vi "Main.vi"(11 "Module Admin":refnum<class "Delacor_lib_QMH_Module Admin.lvclass">) -> ()   [LabVIEW 2020, in "Wordle Engine.lvlib"]
doc: "This template is based off of the Queued Message Handler design pattern and the Queued Message Handler project template that ships with LabVIEW.\n\nThe main difference is that the queue is private to this module and communication between modules is performed via Broadcast and Request events.\n\nRequest events are wrapped in public API methods and are handled in the Event Handling Loop (EHL) of this VI. Any module can register for Broadcast events sent by this module. The EHL generates messages based on user interface actions.\n\nThe Message Handling Loop (MHL) processes messages generated by the EHL, or by other messages. The messages are string values, so new messages can be added easily to the Message Cases case structure in the MHL. Each message cluster can also provide an optional value for Message Data, which is a variant that can be converted to whatever message-specific data is required.\n_____\nBased on DQMH Project Template 6.1.0.93."
uses:
  Wordle Engine.lvlib
  <vilib>/Delacor/Delacor QMH/Libraries/Module Admin_class/Delacor_lib_QMH_Module Admin.lvclass
  Module Data--cluster.ctl
  Stop Argument--cluster.ctl
  <vilib>/Delacor/Delacor QMH/Libraries/Message Queue_class/Delacor_lib_QMH_Message Queue.lvclass/Delacor_lib_QMH_Message Queue.ctl
  <vilib>/Delacor/Delacor QMH/Libraries/Module Admin_class/Delacor_lib_QMH_Module Admin.lvclass/Delacor_lib_QMH_Module Admin.ctl
  Select New Word Argument--cluster.ctl
  Select New Word (Reply Payload)--cluster.ctl
  Make a Guess Argument--cluster.ctl
  Make a Guess (Reply Payload)--cluster.ctl
  Apply Solver Argument--cluster.ctl
  Apply Solver (Reply Payload)--cluster.ctl
  Debug - Solve Specific Word Argument--cluster.ctl
  Debug - Solve Specific Word (Reply Payload)--cluster.ctl
  <vilib>/Delacor/Delacor QMH/Libraries/Message Queue_class/Delacor_lib_QMH_Enqueue Message (Single).vi
  <vilib>/Delacor/Delacor QMH/Libraries/Module Admin_class/Delacor_lib_QMH_Get External Launch.vi
  <vilib>/Utility/error.llb/Error Cluster From Error Code.vi
  <vilib>/ErrorRing/Error Ring.xnode
  <vilib>/Delacor/Delacor QMH/Libraries/Message Queue_class/Delacor_lib_QMH_Message Queue.lvclass
panel:
  out "error out":errorcluster
  # "This is a headless module."
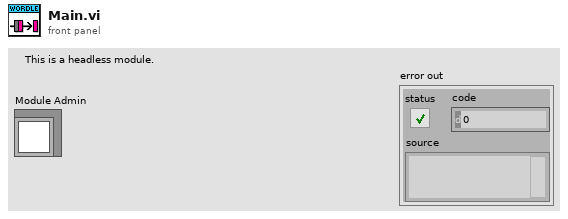
[diagram p1: front panel]
types:
  T1 = typedef "Wordle Engine.lvlib/Request Events--cluster.ctl" = cluster{"Stop Module":refnum<user-event>, "Show Panel":refnum<user-event>, "Hide Panel":refnum<user-event>, "Get Module Execution Status":refnum<user-event>, "Show Diagram":refnum<user-event>, "Select New Word":refnum<user-event>, "Make a Guess":refnum<user-event>, "Apply Solver":refnum<user-event>, "Debug - Solve Specific Word":refnum<user-event>}
  T2 = typedef "Wordle Engine.lvlib/Module Data--cluster.ctl" = cluster{"Used Words":set{string}, "Current Word":string}
  T3 = enum32{"invalid lock state", "Not Locked", "Locked (No Password)", "Password-protected"}
  T4 = typedef "Wordle Engine.lvlib/Stop Argument--cluster.ctl" = cluster{"Origin":string, "Exit via Stop Module Req?":bool, "Wait for Module to stop?":bool}
  T5 = typedef "Wordle Engine.lvlib/Select New Word Argument--cluster.ctl" = cluster{"Exclude Previously Selected Words":bool, "Wait Notifier":refnum<notifier>, "wait for reply":bool}
  T6 = typedef "Wordle Engine.lvlib/Make a Guess Argument--cluster.ctl" = cluster{"Guess":string, "Wait Notifier":refnum<notifier>, "wait for reply":bool}
  T7 = typedef "Wordle Engine.lvlib/Apply Solver Argument--cluster.ctl" = cluster{"Solver VI":path, "Number of Runs (1)":i32, "Wait Notifier":refnum<notifier>, "wait for reply":bool}
  T8 = typedef "Wordle Engine.lvlib/Debug - Solve Specific Word Argument--cluster.ctl" = cluster{"Word to Solve":string, "Solver VI":path, "Wait Notifier":refnum<notifier>, "wait for reply":bool}
  T9 = typedef "Wordle Engine.lvlib/Select New Word (Reply Payload)--cluster.ctl" = cluster{"New Word":string, "error":errorcluster}
  T10 = typedef "Wordle Engine.lvlib/Make a Guess (Reply Payload)--cluster.ctl" = cluster{"Result":string, "error":errorcluster}
  T11 = typedef "Wordle Engine.lvlib/Apply Solver (Reply Payload)--cluster.ctl" = cluster{"Average Solve Count":dbl, "Detailed Results":string, "error":errorcluster}
  T12 = typedef "Wordle Engine.lvlib/Debug - Solve Specific Word (Reply Payload)--cluster.ctl" = cluster{"Results":string, "error":errorcluster}
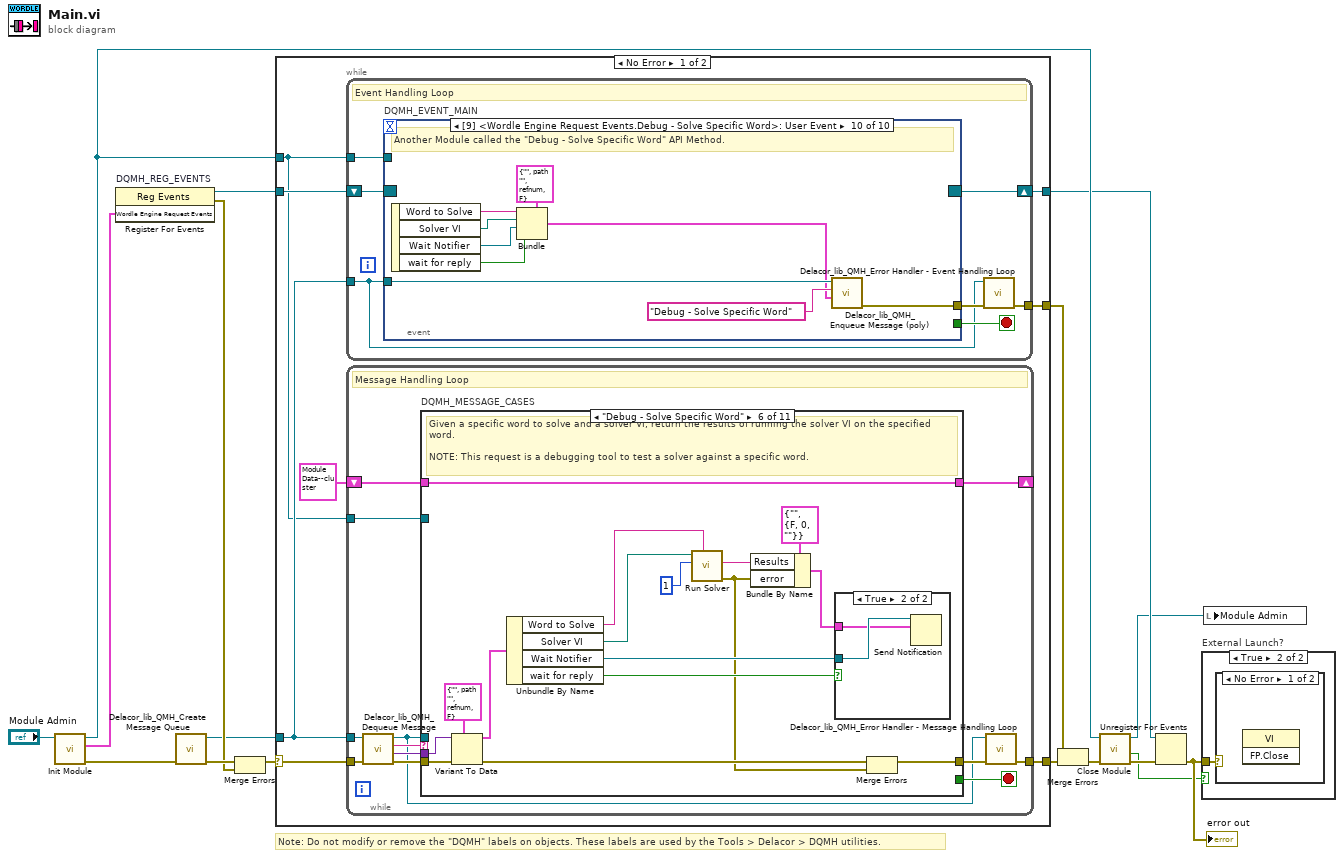
[diagram p0: block diagram]
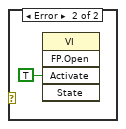
[diagram p3: hidden frame]
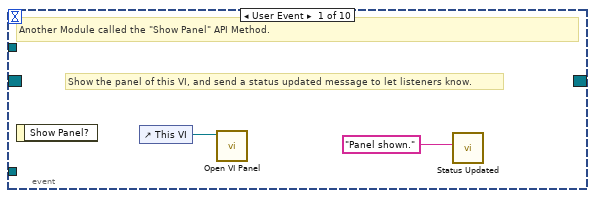
[diagram p4: hidden frame]
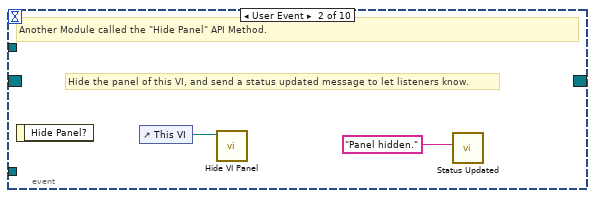
[diagram p5: hidden frame]
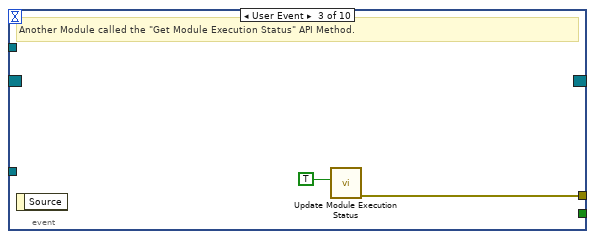
[diagram p6: hidden frame]
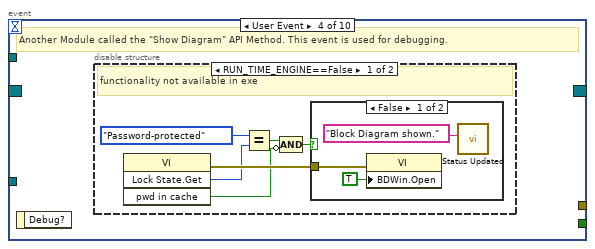
[diagram p7: hidden frame]
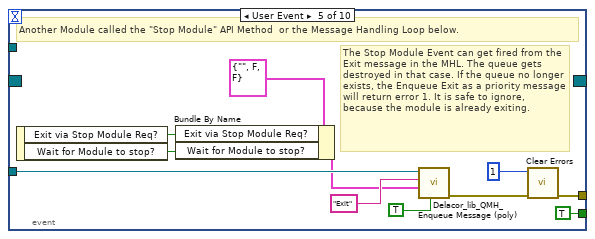
[diagram p10: hidden frame]
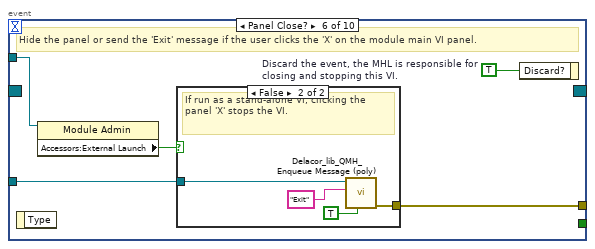
[diagram p11: hidden frame]
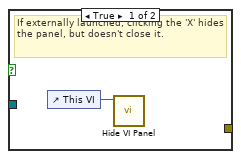
[diagram p12: hidden frame]
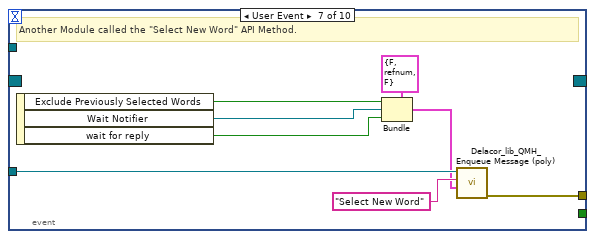
[diagram p13: hidden frame]
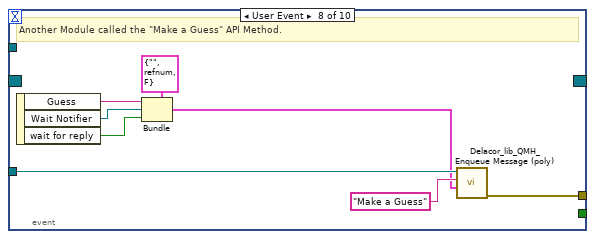
[diagram p14: hidden frame]
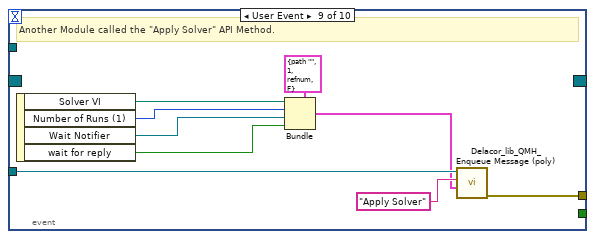
[diagram p15: hidden frame]
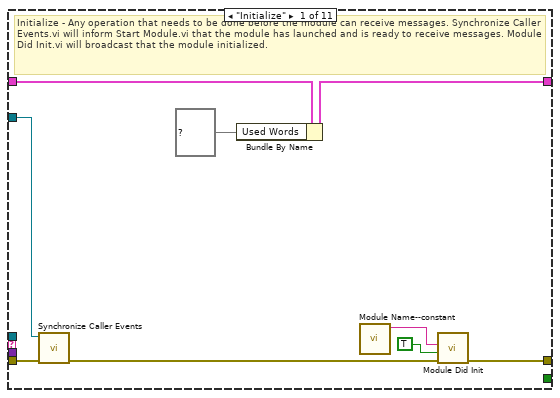
[diagram p16: hidden frame]
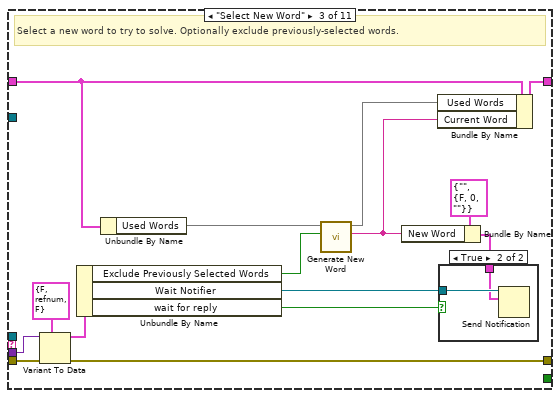
[diagram p18: hidden frame]
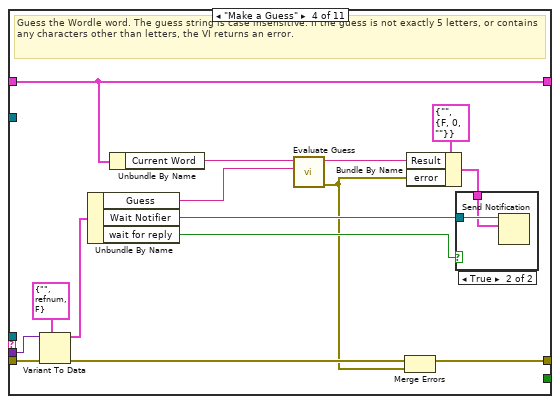
[diagram p20: hidden frame]
diagram:
  # "Note: Do not modify or remove the \"DQMH\" labels on objects. These labels are used by the Tools > Delacor > DQMH utilities."
  n1 = call "Init Module.vi"("Singleton Module Admin in"="Module Admin") -> ("error out"=w16:errorcluster, "Wordle Engine Request Events"=w5:T1, "Singleton Module Admin out"=w8:refnum<class "Delacor_lib_QMH_Module Admin.lvclass">)  [unwired: 8 in]
  n2 = register-events "DQMH_REG_EVENTS"(w5) -> (reference out=w6:refnum<event-registration>, error out=w9:errorcluster)  [unwired: 2 in]
  n3 = call <vilib>:"Delacor_lib_QMH_Create Message Queue.vi"("error in"=w16) -> ("error out"=w11:errorcluster, "Message Queue"=w4:refnum<class "Delacor_lib_QMH_Message Queue.lvclass">)  [unwired: 9 in]
  n4 = Merge Errors(w11, w9) -> (w10:errorcluster)
  n5 = case shown="No Error" w10 {
    selector: w10 -> [w23 w248]
    tunnel: [w25 w247] -> w17
    tunnel: [w22 w253] -> w7
    tunnel: w6 -> [w20 w253]
    tunnel: w4 -> [w19 w246]
    tunnel: [w24 _] -> w14
    tunnel: w8 -> [w18 w249]
    frame No Error {
      n6 = while {
        tunnel: w19 -> [w26]
        shift-right: [w29] -> w22
        shift-left: w20 -> [w30]
        tunnel: [w31] -> w24
        tunnel: w18 -> [w27]
        stop <- w28 stop-if-true
        # "Event Handling Loop"
        n7 = event "DQMH_EVENT_MAIN" shown="[9] <Wordle Engine Request Events.Debug - Solve Specific Word>: User Event" {
          selector: w30 -> [_ _ _ _ _ _ _ _ _ _]
          dyn-events: [_ _ _ _ _ _ _ _ _ _] -> w29
          timeout: _ -> [_ _ _ _ _ _ _ _ _ _]
          tunnel: [_ _ _ _ TRUE ("Discard?") _ _ _ _ _] -> w28
          tunnel: w26 -> [_ _ _ _ w54 w61 w76 w84 w93 w102]
          tunnel: [_ _ w38 _ w57 w63 w69 w77 w85 w94] -> w32
          tunnel: w27 -> [_ _ _ _ _ w60 _ _ _ _]
          event User Event {
            # "Show the panel of this VI, and send a status updated message to let listeners know."
            # "Another Module called the \"Show Panel\" API Method."
            n8 = event-data() -> ()  [unwired: 1 in, 1 out]
            n9 = control-ref of="This VI"() -> (w34:refnum<vi>)
            n10 = call "Open VI Panel.vi"("VI"=w34) -> ()  [unwired: 10 in, 1 out]
            n11 = call "Status Updated.vi"("Status"="Panel shown." ("format string")) -> ()  [unwired: 10 in, 1 out]
          }
          event User Event {
            # "Hide the panel of this VI, and send a status updated message to let listeners know."
            # "Another Module called the \"Hide Panel\" API Method."
            n12 = event-data() -> ()  [unwired: 1 in, 1 out]
            n13 = control-ref of="This VI"() -> (w36:refnum<vi>)
            n14 = call "Hide VI Panel.vi"("VI"=w36) -> ()  [unwired: 10 in, 1 out]
            n15 = call "Status Updated.vi"("Status"="Panel hidden." ("format string")) -> ()  [unwired: 10 in, 1 out]
          }
          event User Event {
            # "Another Module called the \"Get Module Execution Status\" API Method."
            n16 = event-data() -> ()  [unwired: 1 in, 1 out]
            n17 = call "Update Module Execution Status.vi"("Running?"=TRUE) -> ("error out"=w38:errorcluster)  [unwired: 10 in]
          }
          event User Event {
            # "Another Module called the \"Show Diagram\" API Method. This event is used for debugging."
            n18 = event-data() -> ()  [unwired: 1 in, 1 out]
            n19 = disable-structure shown="RUN_TIME_ENGINE==False" {
              frame condition #0 (active) {
                # "functionality not available in exe"
                n20 = invoke class="VI" method="Lock State.Get"() -> (error out=w44:errorcluster, "Get Lock State"=w43:T3, "pwd in cache"=w40:bool)  [unwired: 4 in, 1 out]
                n21 = Equal?(x=T3."Password-protected", y=w43) -> (x = y?=w41:bool)
                n22 = Compound Arithmetic op=AND(w41, invert w40) -> (w39:bool)
                n23 = case shown="False" w39 {
                  tunnel: w44 -> [w47 _]
                  frame False {
                    n24 = property class="VI"(error in=w47, "BDWin.Open"=TRUE ("Block Diagram Window:Open")) -> ()  [unwired: 1 in, 2 out]
                    n25 = call "Status Updated.vi"("Status"="Block Diagram shown." ("format string")) -> ()  [unwired: 10 in, 1 out]
                  }
                  frame True {
                    # "Password-protected VI, and the password is not in the cache. Do not show the diagram."
                  }
                }
              }
              frame condition #1 {
              }
            }
          }
          event User Event {
            # "The Stop Module Event can get fired from the Exit message in the MHL. The queue gets destroyed in that case. If the queue no longer exists, the Enqueue Exit as a priority message will return error 1. It is safe to ignore, because the module is already exiting."
            # "Another Module called the \"Stop Module\" API Method  or the Message Handling Loop below."
            n26 = event-data() -> ("Exit via Stop Module Req?"=w50:bool, "Wait for Module to stop?"=w49:bool)  [unwired: 1 in]
            n27 = Bundle By Name(cluster=T4 {"Origin"="", "Exit via Stop Module Req?"=FALSE, "Wait for Module to stop?"=FALSE} ("Stop Argument"), "Exit via Stop Module Req?"=w50, "Wait for Module to stop?"=w49) -> (w48:T4)
            n28 = call-poly <vilib>:"Delacor_lib_QMH_Enqueue Message (poly).vi"("Priority Message? (F)"=TRUE, "Message Data"=w48, "Message"="Exit", "Message Queue in"=w54) -> ("error out"=w58:errorcluster)  [unwired: 6 in, 1 out]
            n29 = call <vilib>:"Clear Errors.vi"("error in (no error)"=w58, "specific error code to clear (0: all)"=1) -> ("error out"=w57:errorcluster)  [unwired: 4 in, 1 out]
          }
          event Panel Close? {
            w62 = TRUE  # Discard the event, the MHL is responsible for closing and stopping this VI.
            # "Hide the panel or send the 'Exit' message if the user clicks the 'X' on the module main VI panel."
            n30 = event-data() -> ()  [unwired: 1 in, 1 out]
            n31 = property class="Module Admin"(reference=w60) -> ("Accessors:External Launch"=w59:bool)  [unwired: 1 in, 2 out]
            n32 = case shown="False" w59 {
              tunnel: w61 -> [_ w67]
              tunnel: [_ w68] -> w63
              frame True {
                # "If externally launched, clicking the 'X' hides the panel, but doesn't close it."
                n33 = control-ref of="This VI"() -> (w64:refnum<vi>)
                n34 = call "Hide VI Panel.vi"("VI"=w64) -> ()  [unwired: 10 in, 1 out]
              }
              frame False {
                # "If run as a stand-alone VI, clicking the panel 'X' stops the VI."
                n35 = call-poly <vilib>:"Delacor_lib_QMH_Enqueue Message (poly).vi"("Priority Message? (F)"=TRUE, "Message"="Exit", "Message Queue in"=w67) -> ("error out"=w68:errorcluster)  [unwired: 7 in, 1 out]
              }
            }
            n36 = event-data("Discard?"=w62) -> ()  [unwired: 1 in, 1 out]
          }
          event User Event {
            # "Another Module called the \"Select New Word\" API Method."
            n37 = event-data() -> ("Exclude Previously Selected Words"=w72:bool, "Wait Notifier"=w71:refnum<notifier>, "wait for reply"=w70:bool)  [unwired: 1 in]
            n38 = Bundle(cluster=T5 {"Exclude Previously Selected Words"=FALSE, "Wait Notifier"=refnum, "wait for reply"=FALSE} ("Select New Word Argument"), "Exclude Previously Selected Words"=w72, "Wait Notifier"=w71, "wait for reply"=w70) -> (w73:T5)
            n39 = call-poly <vilib>:"Delacor_lib_QMH_Enqueue Message (poly).vi"("Message Data"=w73, "Message"="Select New Word", "Message Queue in"=w76) -> ("error out"=w69:errorcluster)  [unwired: 7 in, 1 out]
          }
          event User Event {
            # "Another Module called the \"Make a Guess\" API Method."
            n40 = event-data() -> ("Guess"=w80:string, "Wait Notifier"=w79:refnum<notifier>, "wait for reply"=w78:bool)  [unwired: 1 in]
            n41 = Bundle(cluster=T6 {"Guess"="", "Wait Notifier"=refnum, "wait for reply"=FALSE} ("Make a Guess Argument"), "Guess"=w80, "Wait Notifier"=w79, "wait for reply"=w78) -> (w81:T6)
            n42 = call-poly <vilib>:"Delacor_lib_QMH_Enqueue Message (poly).vi"("Message Data"=w81, "Message"="Make a Guess", "Message Queue in"=w84) -> ("error out"=w77:errorcluster)  [unwired: 7 in, 1 out]
          }
          event User Event {
            # "Another Module called the \"Apply Solver\" API Method."
            n43 = event-data() -> ("Solver VI"=w89:path, "Number of Runs (1)"=w88:i32, "Wait Notifier"=w87:refnum<notifier>, "wait for reply"=w86:bool)  [unwired: 1 in]
            n44 = Bundle(cluster=T7 {"Solver VI"=path "", "Number of Runs (1)"=1, "Wait Notifier"=refnum, "wait for reply"=FALSE} ("Apply Solver Argument"), "Solver VI"=w89, "Number of Runs (1)"=w88, "Wait Notifier"=w87, "wait for reply"=w86) -> (w90:T7)
            n45 = call-poly <vilib>:"Delacor_lib_QMH_Enqueue Message (poly).vi"("Message Data"=w90, "Message"="Apply Solver", "Message Queue in"=w93) -> ("error out"=w85:errorcluster)  [unwired: 7 in, 1 out]
          }
          event User Event {
            # "Another Module called the \"Debug - Solve Specific Word\" API Method."
            n46 = event-data() -> ("Word to Solve"=w98:string, "Solver VI"=w97:path, "Wait Notifier"=w96:refnum<notifier>, "wait for reply"=w95:bool)  [unwired: 1 in]
            n47 = Bundle(cluster=T8 {"Word to Solve"="", "Solver VI"=path "", "Wait Notifier"=refnum, "wait for reply"=FALSE} ("Debug - Solve Specific Word Argument"), "Word to Solve"=w98, "Solver VI"=w97, "Wait Notifier"=w96, "wait for reply"=w95) -> (w99:T8)
            n48 = call-poly <vilib>:"Delacor_lib_QMH_Enqueue Message (poly).vi"("Message Data"=w99, "Message"="Debug - Solve Specific Word", "Message Queue in"=w102) -> ("error out"=w94:errorcluster)  [unwired: 7 in, 1 out]
          }
        }
        n49 = call-dynamic "Delacor_lib_QMH_Error Handler - Event Handling Loop.vi"("error in"=w32, "Message Queue in"=w26) -> ("dup error in"=w31:errorcluster)  [unwired: 8 in, 1 out]
      }
      n50 = while {
        tunnel: w19 -> [w105]
        shift-right: [w109] -> _
        shift-left: T2 {"Used Words"={}, "Current Word"=""} ("Data Cluster") -> [w110]
        tunnel: w23 -> [w113]
        tunnel: [w111] -> w25
        tunnel: w18 -> [w103]
        stop <- w108 stop-if-true
        # "Message Handling Loop"
        n51 = call-dynamic "Delacor_lib_QMH_Dequeue Message.vi"("error in"=w113, "Message Queue in"=w105) -> ("error out"=w112:errorcluster, "Message Data"=w106:variant, "Message"=w107:string, "Message Queue out"=w104:refnum<class "Delacor_lib_QMH_Message Queue.lvclass">)  [unwired: 6 in]
        n52 = case "DQMH_MESSAGE_CASES" shown="\"Debug - Solve Specific Word\"" w107 {
          selector: w107 -> [_ _ _ _ _ _ _ _ _ _ w233]
          tunnel: w104 -> [_ _ _ _ _ _ _ _ w203 w225 _]
          tunnel: w112 -> [w123 w125 w140 w157 w175 w193 w198 w200 w210 w231 w235]
          tunnel: [w121 w125 w139 w144 w165 w183 w197 w200 w206 w228 w236] -> w114
          tunnel: w110 -> [w119 w124 w129 w148 w174 w192 w196 w199 w205 w224 w234]
          tunnel: [w116 w124 w131 w148 w174 w192 w196 w199 w205 w224 w234] -> w109
          tunnel: [_ _ _ _ _ _ _ _ _ w223 _] -> w108
          tunnel: w106 -> [_ _ w138 w155 w172 w190 _ _ w204 w222 _]
          tunnel: w103 -> [w120 _ _ _ _ _ _ _ w202 w217 _]
          frame "Initialize" {
            # "Initialize - Any operation that needs to be done before the module can receive messages. Synchronize Caller Events.vi will inform Start Module.vi that the module has launched and is ready to receive messages. Module Did Init.vi will broadcast that the module initialized."
            n53 = call "Synchronize Caller Events.vi"("error in (no error)"=w123, "Singleton Module Admin in"=w120) -> ("error out"=w122:errorcluster)  [unwired: 8 in, 1 out]
            n54 = Bundle By Name(cluster=w119, "Used Words"=set{string} {}) -> (w116:T2)
            n55 = call "Module Name--constant.vi"() -> ("Module Name"=w117:string)  [unwired: 11 in]
            n56 = call "Module Did Init.vi"("error in (no error)"=w122, "Initialized?"=TRUE, "Origin"=w117) -> ("error out"=w121:errorcluster)  [unwired: 8 in]
          }
          frame "---Module Specific---" {
            # "Separator -- The following cases handle messages specific to this Module."
          }
          frame "Select New Word" {
            # "Select a new word to try to solve. Optionally exclude previously-selected words."
            n57 = Variant To Data(error in=w140, type=T5 {"Exclude Previously Selected Words"=FALSE, "Wait Notifier"=refnum, "wait for reply"=FALSE} ("Select New Word Argument"), Variant=w138) -> (data=w136:T5, error out=w139:errorcluster)
            n58 = Unbundle By Name(w136) -> ("Exclude Previously Selected Words"=w127:bool, "Wait Notifier"=w135:refnum<notifier>, "wait for reply"=w134:bool)
            n59 = Unbundle By Name(w129) -> ("Used Words"=w128:set{string})
            n60 = call "Generate New Word.vi"("Exclude Previously Selected Words"=w127, "Used Words in"=w128) -> ("Random Element"=w126:string, "Used Words out"=w130:set{string})  [unwired: 8 in]
            n61 = Bundle By Name(cluster=T9 {"New Word"="", "error"={"status"=FALSE, "code"=0, "source"=""}} ("Select New Word (Reply Payload)"), "New Word"=w126) -> (w133:T9)
            n62 = Bundle By Name(cluster=w129, "Used Words"=w130, "Current Word"=w126) -> (w131:T2)
            n63 = case shown="True" w134 {
              tunnel: w135 -> [_ w142]
              tunnel: w133 -> [_ w141]
              frame False {
              }
              frame True {
                n64 = Send Notification(notification=w141, notifier=w142) -> ()  [unwired: 1 in, 2 out]
              }
            }
          }
          frame "Make a Guess" {
            # "Guess the Wordle word. The guess string is case insensitive. If the guess is not exactly 5 letters, or contains any characters other than letters, the VI returns an error."
            n65 = Variant To Data(error in=w157, type=T6 {"Guess"="", "Wait Notifier"=refnum, "wait for reply"=FALSE} ("Make a Guess Argument"), Variant=w155) -> (data=w153:T6, error out=w156:errorcluster)
            n66 = Unbundle By Name(w153) -> ("Guess"=w146:string, "Wait Notifier"=w152:refnum<notifier>, "wait for reply"=w151:bool)
            n67 = Unbundle By Name(w148) -> ("Current Word"=w147:string)
            n68 = call "Evaluate Guess.vi"("Guess"=w146, "Current Word"=w147) -> ("error out"=w143:errorcluster, "Result"=w145:string)  [unwired: 8 in]
            n69 = Merge Errors(w156, w143) -> (w144:errorcluster)
            n70 = Bundle By Name(cluster=T10 {"Result"="", "error"={"status"=FALSE, "code"=0, "source"=""}} ("Make a Guess (Reply Payload)"), "Result"=w145, "error"=w143) -> (w150:T10)
            n71 = case shown="True" w151 {
              tunnel: w152 -> [_ w159]
              tunnel: w150 -> [_ w158]
              frame False {
              }
              frame True {
                n72 = Send Notification(notification=w158, notifier=w159) -> ()  [unwired: 1 in, 2 out]
              }
            }
          }
          frame "Apply Solver" {
            # "Applies a Solver VI to a specified number of Wordle words."
            n73 = Variant To Data(error in=w175, type=T7 {"Solver VI"=path "", "Number of Runs (1)"=1, "Wait Notifier"=refnum, "wait for reply"=FALSE} ("Apply Solver Argument"), Variant=w172) -> (data=w170:T7, error out=w173:errorcluster)
            n74 = Unbundle By Name(w170) -> ("Solver VI"=w164:path, "Number of Runs (1)"=w163:i32, "Wait Notifier"=w169:refnum<notifier>, "wait for reply"=w168:bool)
            n75 = call "Run Solver.vi"("Number of Solves"=w163, "Solver"=w164) -> ("error out"=w160:errorcluster, "Detailed Results"=w161:string, "Average Number of Guesses"=w162:dbl)  [unwired: 7 in]
            n76 = Bundle By Name(cluster=T11 {"Average Solve Count"=0.0, "Detailed Results"="", "error"={"status"=FALSE, "code"=0, "source"=""}} ("Apply Solver (Reply Payload)"), "Average Solve Count"=w162, "Detailed Results"=w161, "error"=w160) -> (w167:T11)
            n77 = case shown="True" w168 {
              tunnel: w169 -> [_ w177]
              tunnel: w167 -> [_ w176]
              frame False {
              }
              frame True {
                n78 = Send Notification(notification=w176, notifier=w177) -> ()  [unwired: 1 in, 2 out]
              }
            }
            n79 = Merge Errors(w173, w160) -> (w165:errorcluster)
          }
          frame "Debug - Solve Specific Word" {
            # "Given a specific word to solve and a solver VI, return the results of running the solver VI on the specified word.\n\nNOTE: This request is a debugging tool to test a solver against a specific word."
            n80 = Variant To Data(error in=w193, type=T8 {"Word to Solve"="", "Solver VI"=path "", "Wait Notifier"=refnum, "wait for reply"=FALSE} ("Debug - Solve Specific Word Argument"), Variant=w190) -> (data=w188:T8, error out=w191:errorcluster)
            n81 = Unbundle By Name(w188) -> ("Word to Solve"=w181:string, "Solver VI"=w180:path, "Wait Notifier"=w187:refnum<notifier>, "wait for reply"=w186:bool)
            n82 = call "Run Solver.vi"("Debug Word (\"\")"=w181, "Number of Solves"=1, "Solver"=w180) -> ("error out"=w179:errorcluster, "Detailed Results"=w182:string)  [unwired: 6 in, 1 out]
            n83 = Bundle By Name(cluster=T12 {"Results"="", "error"={"status"=FALSE, "code"=0, "source"=""}} ("Debug - Solve Specific Word (Reply Payload)"), "Results"=w182, "error"=w179) -> (w185:T12)
            n84 = case shown="True" w186 {
              tunnel: w187 -> [_ w195]
              tunnel: w185 -> [_ w194]
              frame False {
              }
              frame True {
                n85 = Send Notification(notification=w194, notifier=w195) -> ()  [unwired: 1 in, 2 out]
              }
            }
            n86 = Merge Errors(w191, w179) -> (w183:errorcluster)
          }
          frame "---Copy This Frame---" {
            # "Duplicate this frame when creating new messages.  Change this comment in the duplicated frame to describe this message."
            n87 = Merge Errors(w198) -> (w197:errorcluster)
          }
          frame "---Exit and Error Handling---" {
            # "Separator - The following cases handle errors and exit messages."
          }
          frame "Error" {
            # "Error - Check the error message data and respond accordingly. This message is sent by the \"Error Handler\" VIs at the end of each loop in this application."
            n88 = property class="Module Admin"(reference=w202) -> ("Accessors:External Launch"=w201:bool)  [unwired: 1 in, 2 out]
            n89 = Variant To Data(error in=w210, type=errorcluster {"status"=FALSE, "code"=0, "source"=""} ("error constant"), Variant=w204) -> (data=w211:errorcluster, error out=w208:errorcluster)
            n90 = call "Error Reported.vi"("Error"=w211) -> ()  [unwired: 10 in, 1 out]
            n91 = case shown="False" w201 {
              tunnel: [w216 _] -> w207
              tunnel: w203 -> [w214 _]
              tunnel: w211 -> [w215 _]
              frame False {
                # "If the module is running standalone, then pop up an error dialog and call the \"Exit\" message."
                n92 = call <vilib>:"Simple Error Handler.vi"("error in (no error)"=w215) -> ()  [unwired: 4 in, 5 out]
                n93 = call-poly <vilib>:"Delacor_lib_QMH_Enqueue Message (poly).vi"("Priority Message? (F)"=TRUE, "Message"="Exit", "Message Queue in"=w214) -> ("error out"=w216:errorcluster)  [unwired: 7 in, 1 out]
              }
              frame True {
                # "If the module was launched externally, calling the Error Reported broadcast VI is the only action performed by the \"Error\" message. The module's caller can then process the error appropriately."
              }
            }
            n94 = Merge Errors(w208, w207) -> (w206:errorcluster)
            n95 = local write "error out"(w206) -> ()
          }
          frame "Exit" {
            w223 = TRUE  # Stop the VI
            # "Release the message queue reference"
            # "Exit - Exit the application."
            n96 = Variant To Data(error in=w231, type=T4 {"Origin"="", "Exit via Stop Module Req?"=FALSE, "Wait for Module to stop?"=FALSE} ("Stop Argument"), Variant=w222) -> (data=w219:T4, error out=w227:errorcluster)
            n97 = call <vilib>:"Clear Errors.vi"("error in (no error)"=w227, "specific error code to clear (0: all)"=91 ("91: not all Exit messages will have an argument")) -> ("error out"=w230:errorcluster)  [unwired: 4 in, 1 out]
            n98 = control-ref of="This VI"() -> (w218:refnum<vi>)
            n99 = call-dynamic "Delacor_lib_QMH_Release Message Queue.vi"("error in"=w230, "Message Queue"=w225) -> ("error out"=w229:errorcluster)  [unwired: 9 in]
            n100 = call "Handle Exit.vi"("Stop Argument"=w219, "Admin in"=w217, "VI reference"=w218) -> ("error out"=w226:errorcluster)  [unwired: 7 in, 1 out]
            n101 = Merge Errors(w229, w226) -> (w228:errorcluster)
          }
          frame Default {
            # "'Default' case only runs if there is a message that isn't defined in any of the other cases.  Output a programming error."
            n102 = call "Module Name--constant.vi"() -> ("Module Name"=w232:string)  [unwired: 11 in]
            n103 = xnode "Error Ring"("parameter 0"=w233, "parameter 1"=w232) -> ("error out"=w237:errorcluster)
            n104 = Merge Errors(w235, w237) -> (w236:errorcluster)
          }
        }
        n105 = call-dynamic "Delacor_lib_QMH_Error Handler - Message Handling Loop.vi"("error in"=w114, "Message Queue in"=w104) -> ("dup error in"=w111:errorcluster)  [unwired: 8 in, 1 out]
      }
    }
    frame Error {
      # "Synchronize Caller Events.vi will inform Start Module.vi that the module has launched and will let the code calling Start Module.vi register for broadcasts and would permit the caller receive the broadcast that an error occurred at launch time."
      n106 = call-dynamic "Delacor_lib_QMH_Release Message Queue.vi"("error in"=w248, "Message Queue"=w246) -> ("error out"=w247:errorcluster)  [unwired: 9 in]
      n107 = call "Synchronize Caller Events.vi"("Singleton Module Admin in"=w249) -> ("error out"=w254:errorcluster)  [unwired: 9 in, 1 out]
      n108 = call "Module Name--constant.vi"() -> ("Module Name"=w252:string)  [unwired: 11 in]
      n109 = Format Into String(format string="An error occurred during initialization. %s is no longer running.", w252) -> (resulting string=w250:string)  [unwired: 2 in, 1 out]
      n110 = Merge Errors(w247, w254) -> (w255:errorcluster)
      n111 = call "Error Reported.vi"("Additional Information"=w250, "Error"=w255) -> ()  [unwired: 9 in, 1 out]
    }
  }
  n112 = Merge Errors(w14, w17) -> (w13:errorcluster)
  n113 = call "Close Module.vi"("error in (no error)"=w13, "Module Admin in"=w8) -> ("error out"=w15:errorcluster, "External Launch"=w1:bool, "Module Admin out"=w2:refnum<class "Delacor_lib_QMH_Module Admin.lvclass">)  [unwired: 7 in]
  n114 = Unregister For Events(event registration refnum=w7, error in=w15) -> (error out=w12:errorcluster)
  "error out" <- w12
  n115 = case "External Launch?" shown="True" w1 {
    tunnel: w12 -> [_ w256]
    frame False {
    }
    frame True {
      n116 = case shown="No Error" w256 {
        frame No Error {
          n117 = invoke class="VI" method="FP.Close"() -> ()  [unwired: 3 in, 3 out]
        }
        frame Error {
          n118 = invoke class="VI" method="FP.Open"("Activate"=TRUE ("Activate?")) -> ()  [unwired: 4 in, 5 out]
        }
      }
    }
  }
  n119 = local write "Module Admin"(w2) -> ()
